vi "Reflex_Tester_Final.vi"() -> ()   [LabVIEW 2019]
uses:
  States.ctl
  Results.ctl
  <vilib>/Analysis/NI_AALBase.lvlib
panel:
  in  "stop":bool
  in  "Next Round":bool
  out "Info":string
  out "Best response time:":dbl
  out "Worst response time:":dbl
  in  "Reset":bool
  out "Median response time:":dbl
  out "Last-5":dbl
  out "Last-4":dbl
  out "Last-3":dbl
  out "Last-2":dbl
  out "Last-1":dbl
  out "Last":dbl
  out "Average response time:":dbl
  out "Wrong choices:":u16
  out "Instructions":string
  out "Invalid Tests:":u16
  out "Shape":string
  out "Color":string
  in  "RedSquare":bool
  in  "GreenSquare":bool
  in  "GreenCircle":bool
  in  "RedCircle":bool
  # "Latest Results"
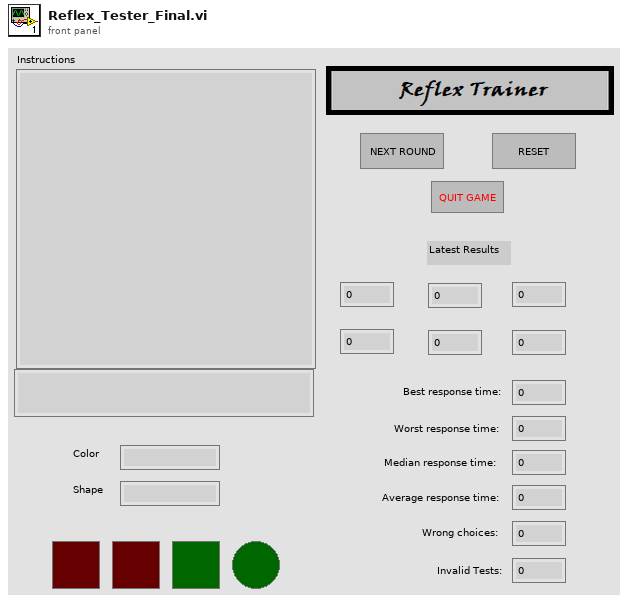
[diagram p1: front panel]
types:
  T1 = typedef "Results.ctl" = cluster{"Wrongs":u16, "Invalids":u16, "Times":dbl[], "Valids":u32, "TotalSum":ext, "Best":dbl, "Worst":dbl}
  T2 = typedef "States.ctl" = enum16{"EndGame", "PlayRound", "Start", "ShowStats", "PrepareNextRound"}
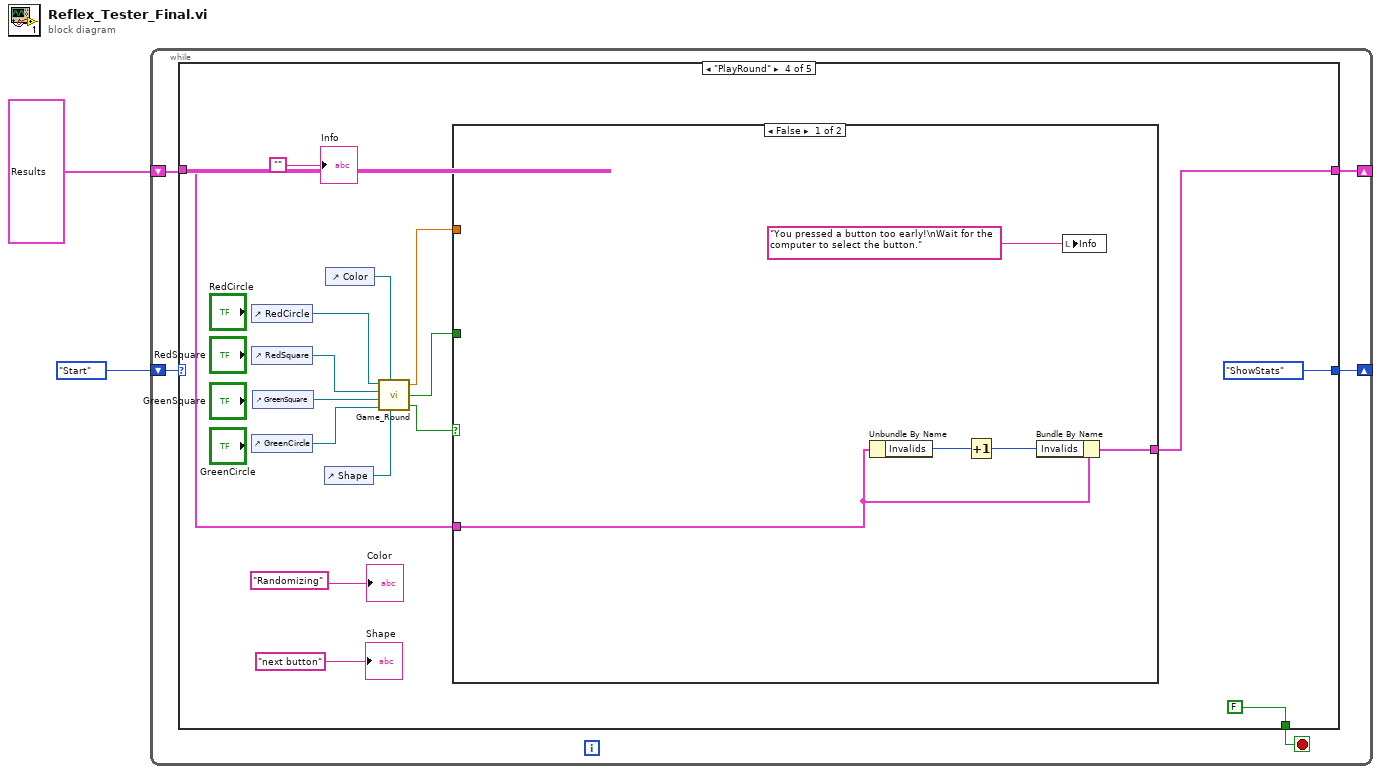
[diagram p0: block diagram]
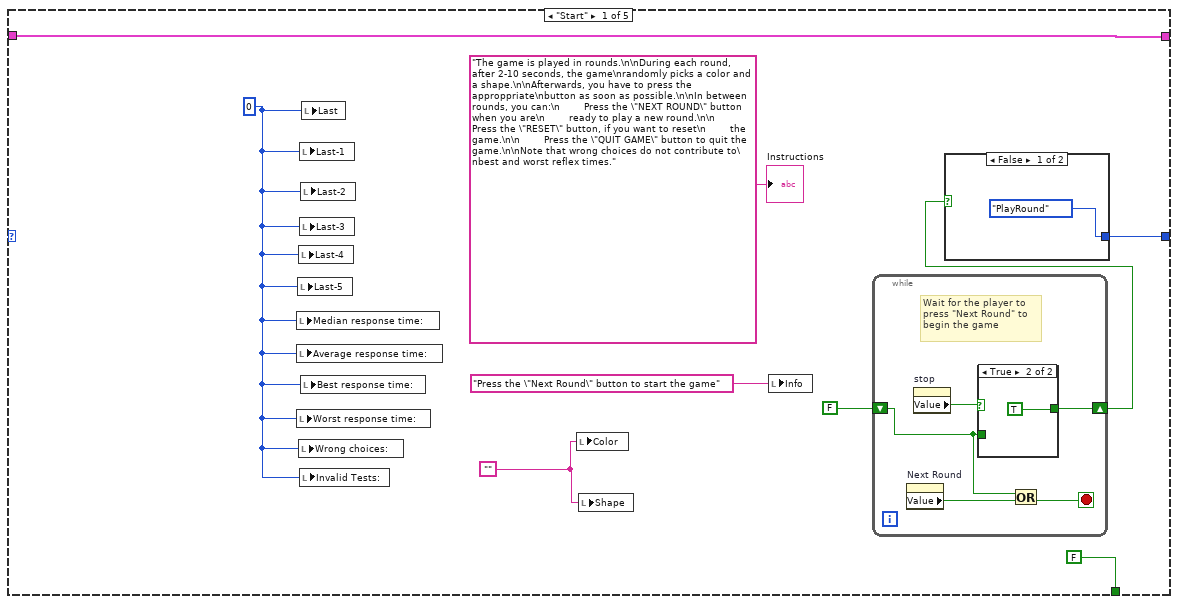
[diagram p2: hidden frame]
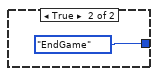
[diagram p3: hidden frame]
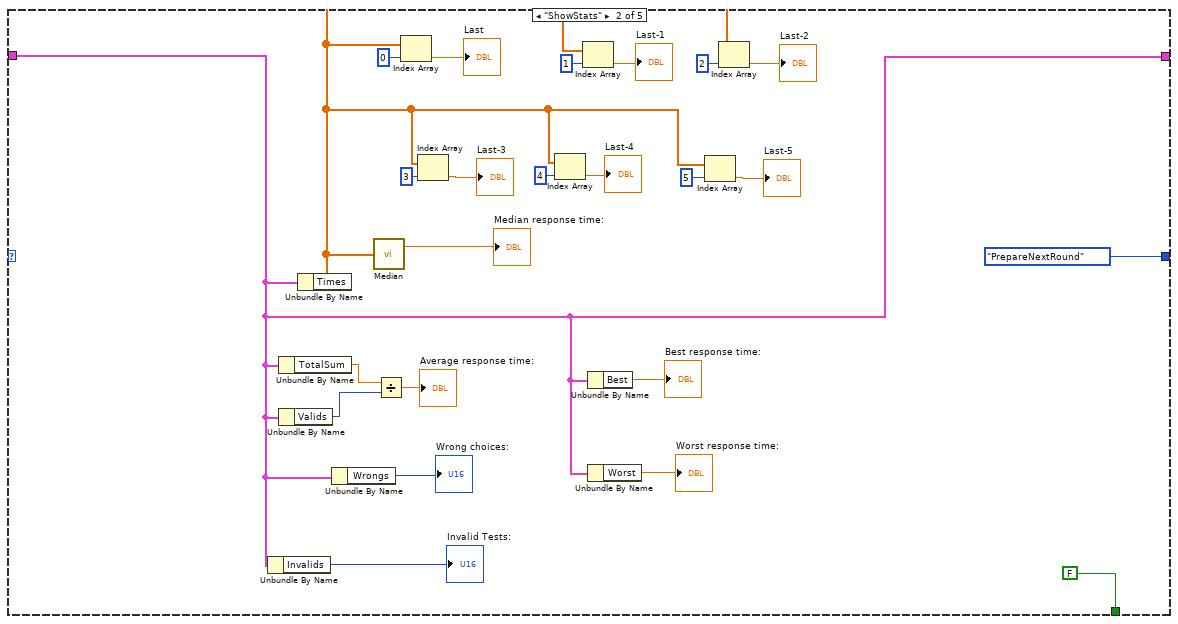
[diagram p5: hidden frame]
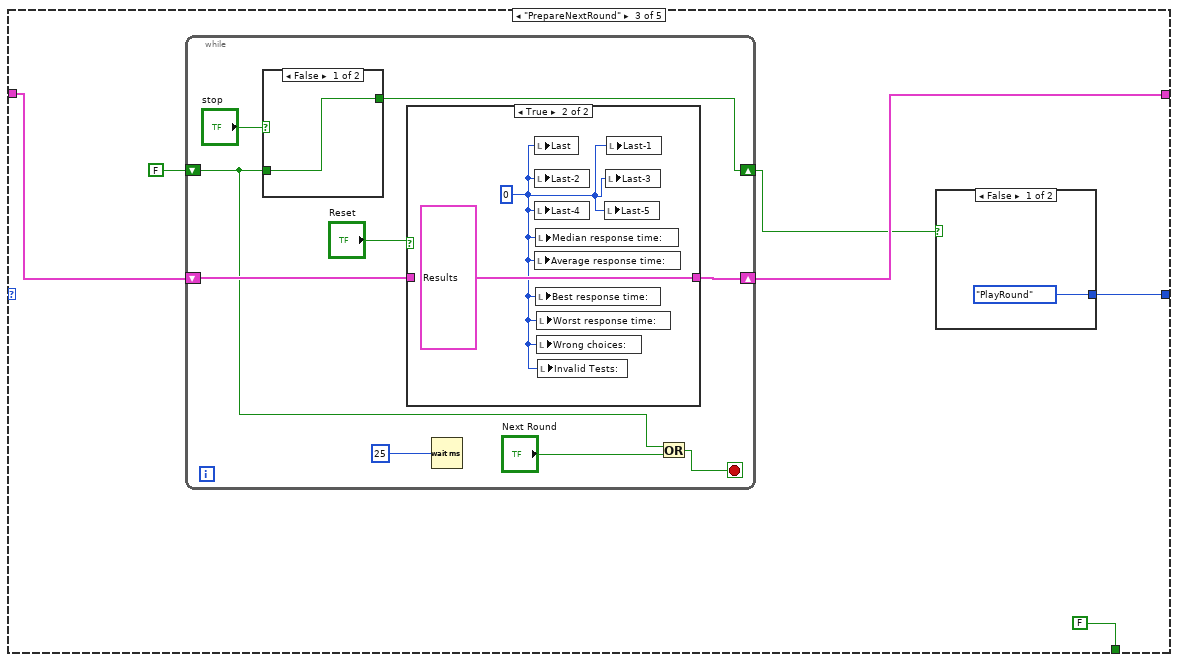
[diagram p6: hidden frame]
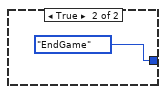
[diagram p7: hidden frame]
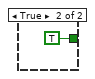
[diagram p8: hidden frame]
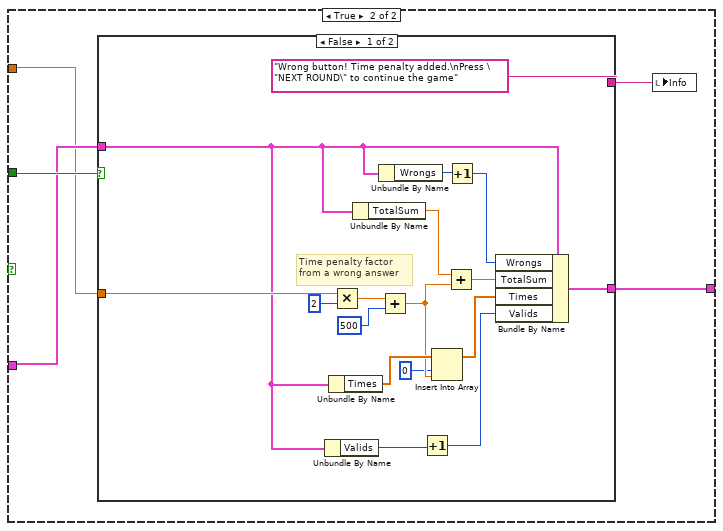
[diagram p10: hidden frame]
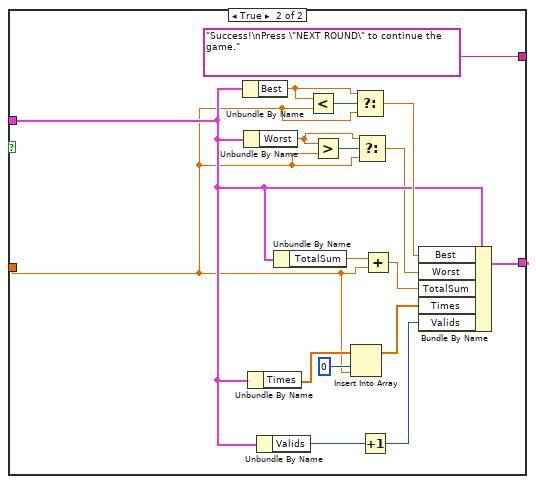
[diagram p11: hidden frame]
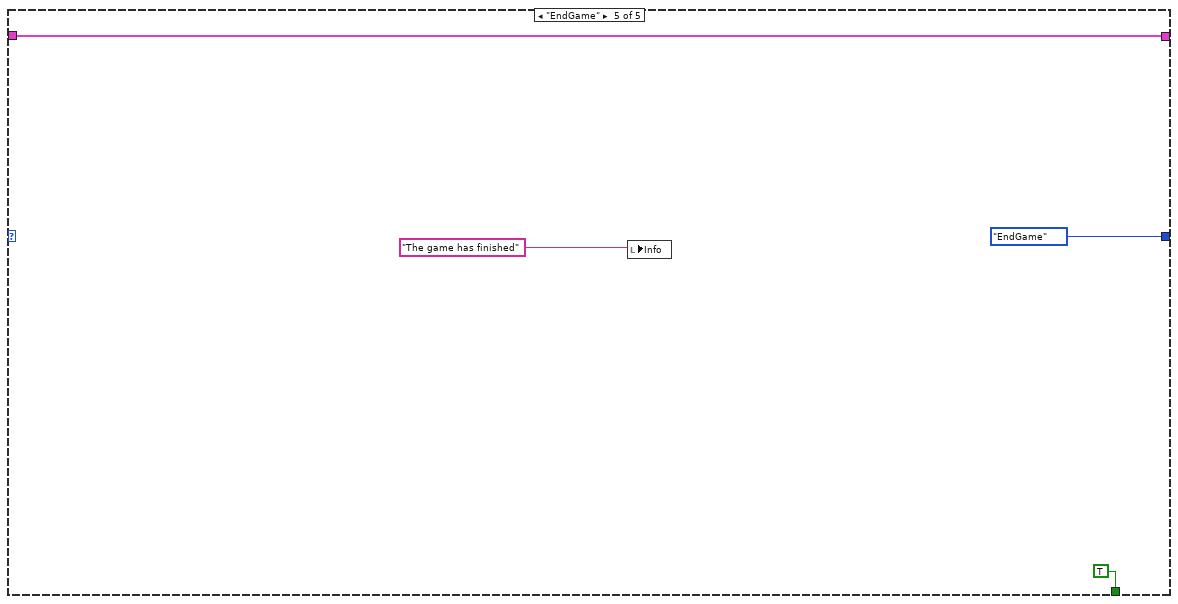
[diagram p12: hidden frame]
diagram:
  n1 = while {
    shift-right: [w4] -> _
    shift-left: T1 {"Wrongs"=0, "Invalids"=0, "Times"=[], "Valids"=0, "TotalSum"=0.0, "Best"=0.0, "Worst"=0.0} ("Results") -> [w6]
    shift-right: [w5] -> _
    shift-left: States."Start" -> [w7]
    stop <- w3 stop-if-true
    n2 = case shown="\"PlayRound\"" w7 {
      tunnel: w6 -> [w12 w28 w55 w81 w133]
      tunnel: [w13 States."PrepareNextRound" ("Enum") w51 States."ShowStats" ("Enum") States."EndGame" ("Enum")] -> w5
      tunnel: [w12 w28 w54 w77 w133] -> w4
      tunnel: [FALSE FALSE FALSE FALSE TRUE] -> w3
      frame "Start" {
        w8 = 0
        w14 = ""
        n3 = local write "Median response time:"(w8) -> ()
        n4 = local write "Average response time:"(w8) -> ()
        n5 = local write "Worst response time:"(w8) -> ()
        n6 = local write "Last-5"(w8) -> ()
        n7 = local write "Last-4"(w8) -> ()
        n8 = local write "Wrong choices:"(w8) -> ()
        n9 = local write "Last-1"(w8) -> ()
        n10 = local write "Last-3"(w8) -> ()
        n11 = local write "Invalid Tests:"(w8) -> ()
        n12 = local write "Last-2"(w8) -> ()
        n13 = local write "Best response time:"(w8) -> ()
        n14 = local write "Last"(w8) -> ()
        n15 = local write "Color"(w14) -> ()
        n16 = local write "Shape"(w14) -> ()
        n17 = local write "Info"("Press the \"Next Round\" button to start the game") -> ()
        n18 = while {
          shift-right: [w22] -> w9
          shift-left: FALSE -> [w19]
          stop <- w21 stop-if-true
          # "Wait for the player to\npress \"Next Round\" to\nbegin the game"
          n19 = property on="Next Round" class="Bool (strict)"() -> ("Value"=w20:bool)  [unwired: 2 in, 2 out]
          n20 = property on="stop" class="Bool (strict)"() -> ("Value"=w23:bool)  [unwired: 2 in, 2 out]
          n21 = case shown="True" w23 {
            tunnel: w19 -> [w24 _]
            tunnel: [w24 TRUE] -> w22
            frame False {
            }
            frame True {
            }
          }
          n22 = Or(x=w19, y=w20) -> (x .or. y?=w21:bool)
        }
        n23 = case shown="False" w9 {
          tunnel: [States."PlayRound" ("Enum") States."EndGame" ("Enum")] -> w13
          frame False {
          }
          frame True {
          }
        }
        "Instructions" <- "The game is played in rounds.\n\nDuring each round, after 2-10 seconds, the game\nrandomly picks a color and a shape.\n\nAfterwards, you have to press the approppriate\nbutton as soon as possible.\n\nIn between rounds, you can:\n        Press the \"NEXT ROUND\" button when you are\n        ready to play a new round.\n\n        Press the \"RESET\" button, if you want to reset\n        the game.\n\n        Press the \"QUIT GAME\" button to quit the game.\n\nNote that wrong choices do not contribute to\nbest and worst reflex times."
      }
      frame "ShowStats" {
        n24 = Unbundle By Name(w28) -> ("Invalids"=→"Invalid Tests:":u16)
        n25 = Unbundle By Name(w28) -> ("TotalSum"=w49:ext)
        n26 = Unbundle By Name(w28) -> ("Valids"=w48:u32)
        n27 = Unbundle By Name(w28) -> ("Times"=w41:dbl[])
        n28 = Unbundle By Name(w28) -> ("Wrongs"=→"Wrong choices:":u16)
        n29 = call <vilib>:"Median.vi"("X"=w41) -> ("median"=→"Median response time:":dbl)  [unwired: 1 out]
        n30 = Divide(x=w49, y=w48) -> (x/y=→"Average response time:":ext)
        n31 = Index Array(array=w41, index=0) -> (element=→"Last":dbl)
        n32 = Index Array(array=w41, index=3) -> (element=→"Last-3":dbl)
        n33 = Index Array(array=w41, index=4) -> (element=→"Last-4":dbl)
        n34 = Index Array(array=w41, index=1) -> (element=→"Last-1":dbl)
        n35 = Unbundle By Name(w28) -> ("Best"=→"Best response time:":dbl)
        n36 = Unbundle By Name(w28) -> ("Worst"=→"Worst response time:":dbl)
        n37 = Index Array(array=w41, index=5) -> (element=→"Last-5":dbl)
        n38 = Index Array(array=w41, index=2) -> (element=→"Last-2":dbl)
      }
      frame "PrepareNextRound" {
        n39 = while {
          shift-right: [w65] -> w54
          shift-left: w55 -> [w66]
          shift-right: [w61] -> w52
          shift-left: FALSE -> [w58]
          stop <- w60 stop-if-true
          n40 = case shown="False" "stop" {
            tunnel: w58 -> [w67 _]
            tunnel: [w67 TRUE] -> w61
            frame False {
            }
            frame True {
            }
          }
          n41 = case shown="True" "Reset" {
            tunnel: w66 -> [w69 _]
            tunnel: [w69 T1 {"Wrongs"=0, "Invalids"=0, "Times"=[], "Valids"=0, "TotalSum"=0.0, "Best"=nan, "Worst"=nan} ("Results")] -> w65
            frame False {
            }
            frame True {
              w70 = 0
              n42 = local write "Last"(w70) -> ()
              n43 = local write "Last-2"(w70) -> ()
              n44 = local write "Last-4"(w70) -> ()
              n45 = local write "Average response time:"(w70) -> ()
              n46 = local write "Median response time:"(w70) -> ()
              n47 = local write "Best response time:"(w70) -> ()
              n48 = local write "Worst response time:"(w70) -> ()
              n49 = local write "Wrong choices:"(w70) -> ()
              n50 = local write "Invalid Tests:"(w70) -> ()
              n51 = local write "Last-5"(w70) -> ()
              n52 = local write "Last-3"(w70) -> ()
              n53 = local write "Last-1"(w70) -> ()
            }
          }
          n54 = Wait (ms)(milliseconds to wait=25) -> ()  [unwired: 1 out]
          n55 = Or(x=w58, y="Next Round") -> (x .or. y?=w60:bool)
        }
        n56 = case shown="False" w52 {
          tunnel: [States."PlayRound" ("Enum") States."EndGame" ("Enum")] -> w51
          frame False {
          }
          frame True {
          }
        }
      }
      frame "PlayRound" {
        n57 = control-ref of="RedCircle"() -> (w87:refnum<vi>)
        n58 = control-ref of="RedSquare"() -> (w86:refnum<vi>)
        n59 = control-ref of="GreenCircle"() -> (w84:refnum<vi>)
        n60 = control-ref of="GreenSquare"() -> (w85:refnum<vi>)
        n61 = control-ref of="Shape"() -> (w83:refnum<vi>)
        n62 = control-ref of="Color"() -> (w82:refnum<vi>)
        n63 = call "Game_Round.vi"("Red Circle"=w87, "ColorStr"=w82, "Red Square"=w86, "GreenSquare"=w85, "ShapeStr"=w83, "Green Circle"=w84) -> ("Elapsed Time"=w79:dbl, "Correct Answer"=w78:bool, "Valid Answer"=w80:bool)
        n64 = case shown="False" w80 {
          tunnel: w78 -> [_ w97]
          tunnel: w79 -> [_ w94]
          tunnel: w81 -> [w90 w96]
          tunnel: [w89 w95] -> w77
          frame False {
            n65 = Unbundle By Name(w90) -> ("Invalids"=w92:u16)
            n66 = Increment(x=w92) -> (x+1=w91:u16)
            n67 = Bundle By Name(cluster=w90, "Invalids"=w91) -> (w89:T1)
            n68 = local write "Info"("You pressed a button too early!\nWait for the computer to select the button.") -> ()
          }
          frame True {
            n69 = case shown="False" w97 {
              tunnel: ["Wrong button! Time penalty added.\nPress \"NEXT ROUND\" to continue the game" "Success!\nPress \"NEXT ROUND\" to continue the game."] -> w93
              tunnel: w96 -> [w104 w120]
              tunnel: [w111 w124] -> w95
              tunnel: w94 -> [w110 w115]
              frame False {
                # "Time penalty factor\nfrom a wrong answer"
                n70 = Unbundle By Name(w104) -> ("Valids"=w99:u32)
                n71 = Unbundle By Name(w104) -> ("Times"=w103:dbl[])
                n72 = Multiply(x=w110, y=2) -> (x*y=w107:dbl)
                n73 = Unbundle By Name(w104) -> ("TotalSum"=w105:ext)
                n74 = Unbundle By Name(w104) -> ("Wrongs"=w112:u16)
                n75 = Add(x=w107, y=500) -> (x+y=w102:dbl)
                n76 = Increment(x=w99) -> (x+1=w98:u32)
                n77 = Insert Into Array(array=w103, index=0, new element=w102) -> (w101:dbl[])
                n78 = Add(x=w105, y=w102) -> (x+y=w106:ext)
                n79 = Increment(x=w112) -> (x+1=w113:u16)
                n80 = Bundle By Name(cluster=w104, "Wrongs"=w113, "TotalSum"=w106, "Times"=w101, "Valids"=w98) -> (w111:T1)
              }
              frame True {
                n81 = Unbundle By Name(w120) -> ("Best"=w117:dbl)
                n82 = Unbundle By Name(w120) -> ("Worst"=w116:dbl)
                n83 = Unbundle By Name(w120) -> ("Times"=w129:dbl[])
                n84 = Unbundle By Name(w120) -> ("Valids"=w126:u32)
                n85 = Unbundle By Name(w120) -> ("TotalSum"=w130:ext)
                n86 = Less?(x=w117, y=w115) -> (x < y?=w123:bool)
                n87 = Greater?(x=w116, y=w115) -> (0:w119:bool)
                n88 = Insert Into Array(array=w129, index=0, new element=w115) -> (w127:dbl[])
                n89 = Select(t=w117, s=w123, f=w115) -> (s? t:f=w121:dbl)
                n90 = Select(t=w116, s=w119, f=w115) -> (s? t:f=w118:dbl)
                n91 = Increment(x=w126) -> (x+1=w125:u32)
                n92 = Add(x=w130, y=w115) -> (x+y=w122:ext)
                n93 = Bundle By Name(cluster=w120, "Best"=w121, "Worst"=w118, "TotalSum"=w122, "Times"=w127, "Valids"=w125) -> (w124:T1)
              }
            }
            n94 = local write "Info"(w93) -> ()
          }
        }
        "Info" <- ""
        "Shape" <- "next button"
        "Color" <- "Randomizing"
      }
      frame "EndGame" {
        n95 = local write "Info"("The game has finished") -> ()
      }
    }
  }
